vi "Write Handle.vi"(8 "error in (no error)":errorcluster, 10 "Handle":string, 11 "NISTFGenPluginsBase in":refnum<class "NISTFGenPluginsBase.lvclass">) -> (0 "error out":errorcluster, 3 "NISTFGenPluginsBase out":refnum<class "NISTFGenPluginsBase.lvclass">)   [LabVIEW 2014, in "FGenPlugins.lvlib" / "NISTFGenPluginsBase.lvclass"]
uses:
  NISTFGenPluginsBase.lvclass
  NISTFGenPluginsBase.lvclass/NISTFGenPluginsBase.ctl
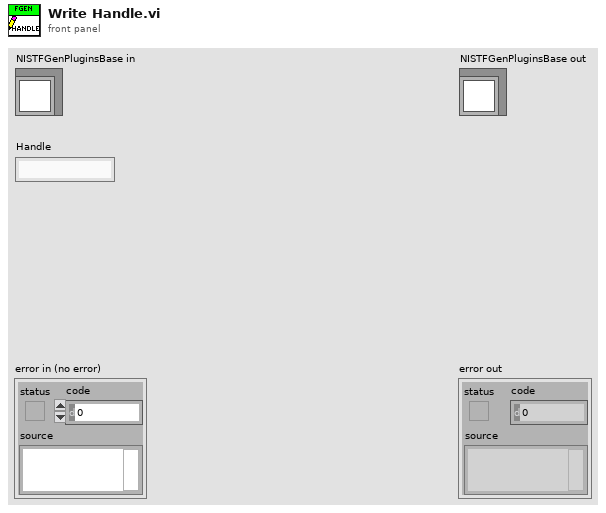
[diagram p1: front panel]
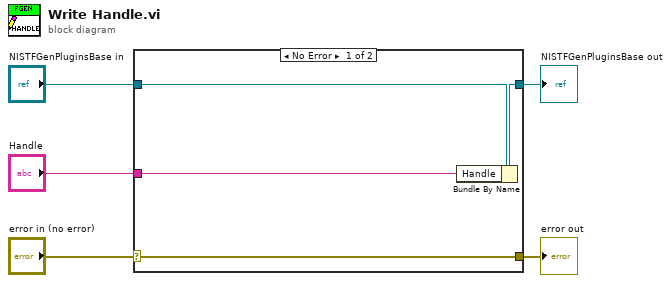
[diagram p0: block diagram]
diagram:
  n1 = case shown="No Error" "error in (no error)" {
    selector: "error in (no error)" -> [w9 w10]
    tunnel: [w9 w10] -> w4
    tunnel: [w7 w11] -> w2
    tunnel: "NISTFGenPluginsBase in" -> [w8 w11]
    tunnel: "Handle" -> [w6 _]
    frame No Error {
      n2 = Bundle By Name(cluster=w8, "Handle"=w6) -> (w7:refnum<class "NISTFGenPluginsBase.lvclass">)
    }
    frame Error {
    }
  }
  "error out" <- w4
  "NISTFGenPluginsBase out" <- w2
